vi "Configure Sample.vi"(8 "error in (no error)":errorcluster, 9 "Sample Timer (1 s)":dbl=1.0, 10 "Sample Count (1)":i32=1, 11 "VISA resource name":refnum<visa-resource-name>) -> (0 "error out":errorcluster, 3 "VISA resource name out":refnum<visa-resource-name>)   [LabVIEW 2020, in "Agilent 34405.lvlib"]
doc: "Configure the sample settings on the instrument.\n\n<B>Notes:</B> \n(1) Use this VI only with other low-level VIs. The high-level VIs automatically incorporate this functionality.\n(2) This VI only support <B>Agilent 34450A</B>."
uses:
  <instrlib>/Agilent 34405/Agilent 34405.lvlib
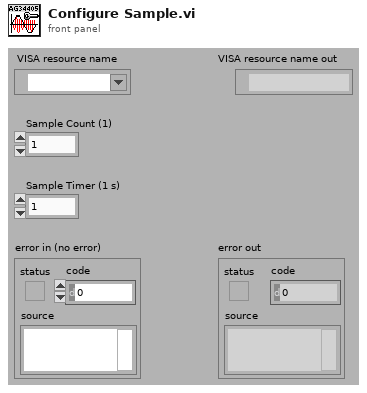
[diagram p1: front panel]
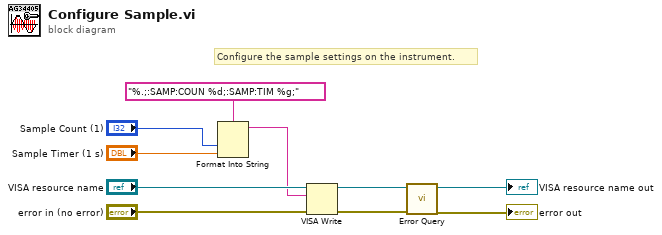
[diagram p0: block diagram]
diagram:
  # "Configure the sample settings on the instrument."
  n1 = Format Into String(format string="%.;:SAMP:COUN %d;:SAMP:TIM %g;", "Sample Count (1)", "Sample Timer (1 s)") -> (resulting string=w1:string)  [unwired: 2 in, 1 out]
  n2 = VISA Write(VISA resource name="VISA resource name", write buffer=w1, error in (no error)="error in (no error)") -> (VISA resource name out=w8:refnum<visa-resource-name>, error out=w7:errorcluster)  [unwired: 1 out]
  n3 = call <instrlib>:"Error Query.vi"("error in (no error)"=w7, "VISA resource name"=w8) -> ("error out"=→"error out":errorcluster, "VISA resource name out"=→"VISA resource name out":refnum<visa-resource-name>)  [unwired: 8 out]
